vi "Loop_HW.vi"() -> ()   [LabVIEW 2017, in "LED Signal.lvlib"]
uses:
  LED Signal.lvlib
  Globals/Global_STOP.vi
  Global_SM_Data Out.vi
  ENUM_HW LED Commands.ctl
  Globals/Global_HW_Address_Assignments.vi
  <vilib>/Rock Robotics/WPI/SerialPort/WPI_SerialPortRef.ctl
  <vilib>/Rock Robotics/WPI/SerialPort/WPI_SerialPort.ctl
  Cluster_SM to HW Data.ctl
panel:
  out "SM LED_HW Cmd Data":T1
  out "SerialPortRef":T4
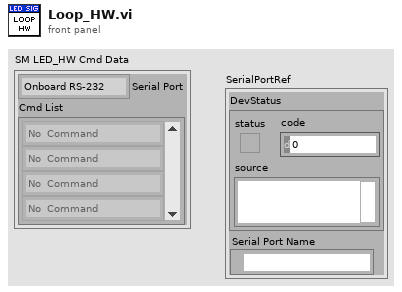
[diagram p1: front panel]
types:
  T1 = typedef "LED Signal.lvlib/Cluster_SM to HW Data.ctl" = cluster{"Serial Port":T2, "Cmd List":T3[]}
  T2 = typedef "WPI_SerialPort.ctl" = enum16{"Onboard RS-232", "MXP TTL", "USB 1", "USB 2"}
  T3 = typedef "LED Signal.lvlib/ENUM_HW LED Commands.ctl" = enum16{"No  Command", "Angled Drive; A", "Field Oriented Drive; D", "Normal Drive; d", "Camera Lined Up; C", "Camera Misallined; c", "Balls in Hopper; B", "Hopper Empty; b"}
  T4 = typedef "WPI_SerialPortRef.ctl" = cluster{"DevStatus":errorcluster, "Serial Port Name":refnum<visa-resource-name>}
  T5 = cluster{"Serial Port":T2, "Baud Rate":u32, "Data Bits":u16, "Parity":u16, "Stop Bits":u16, "Flow Control":u16}
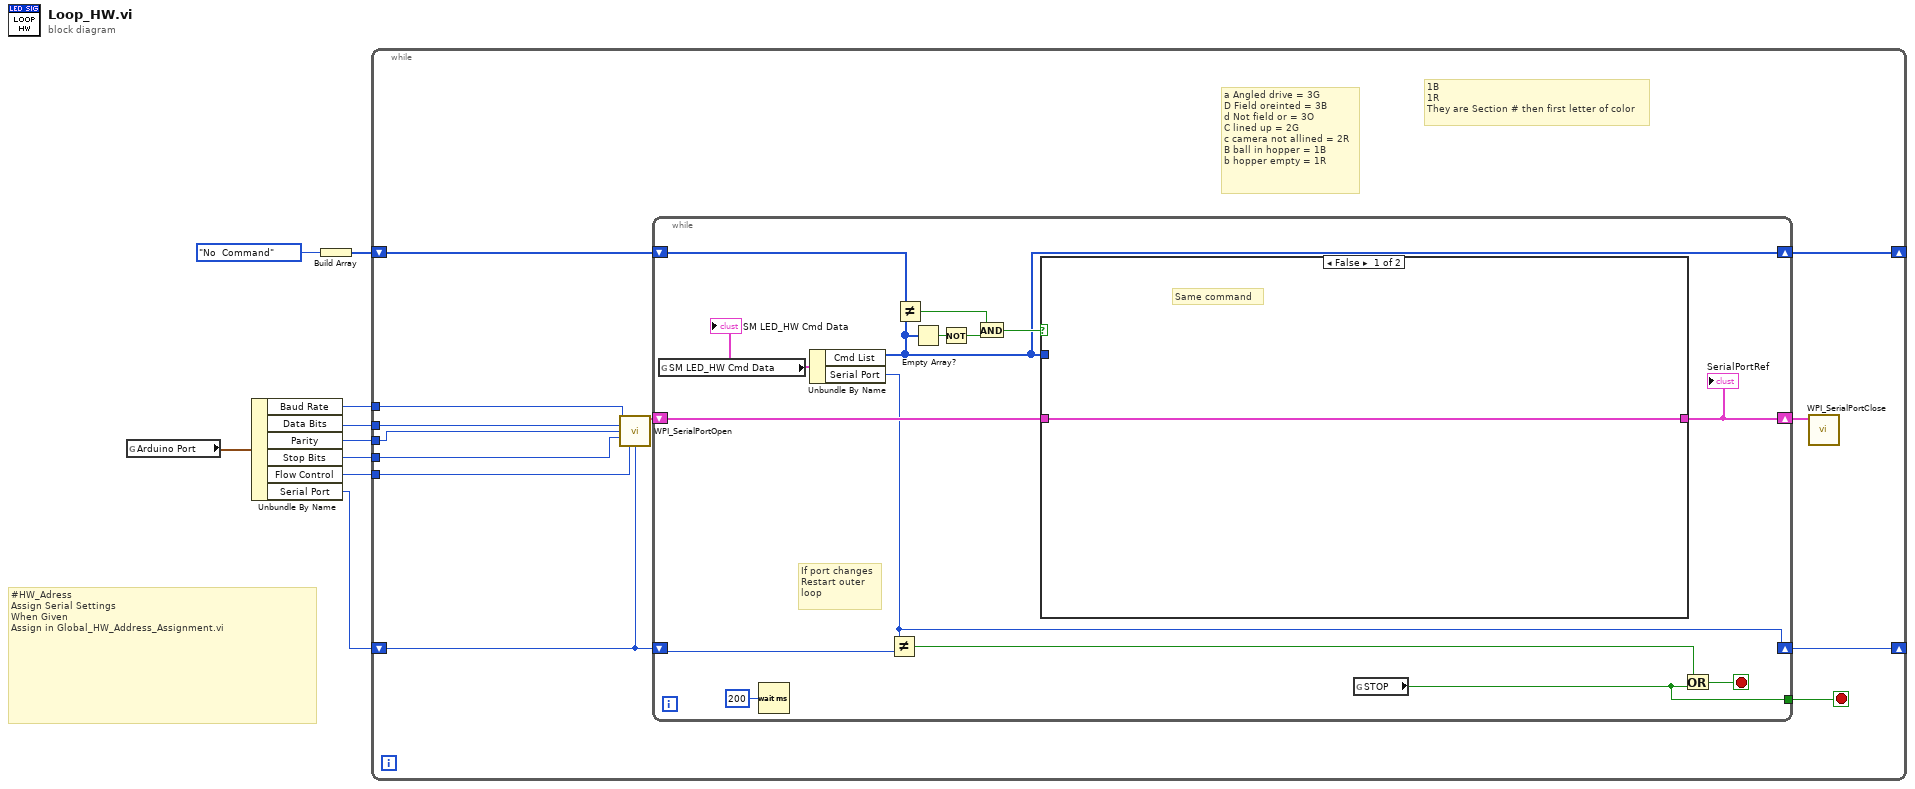
[diagram p0: block diagram]
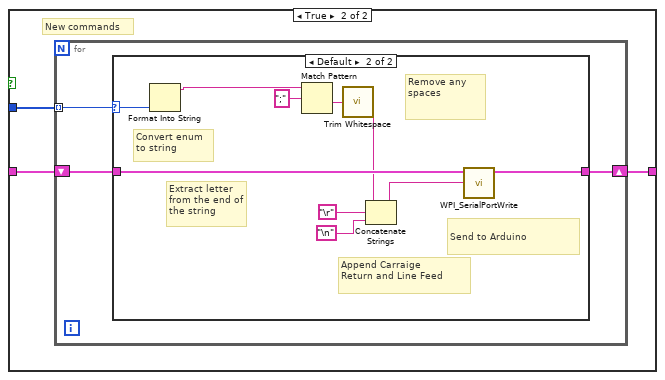
[diagram p2: hidden frame]
diagram:
  # "#HW_Adress\nAssign Serial Settings\nWhen Given\nAssign in Global_HW_Address_Assignment.vi"
  n1 = global read "Global_HW_Address_Assignments.vi" "Arduino Port"() -> (w7:T5)
  n2 = Unbundle By Name(w7) -> ("Baud Rate"=w5:u32, "Data Bits"=w4:u16, "Parity"=w3:u16, "Stop Bits"=w2:u16, "Flow Control"=w1:u16, "Serial Port"=w6:T2)
  n3 = Build Array(ENUM_HW_LED_Commands."No  Command" ("Cmd")) -> (w8:T3[])
  n4 = while {
    shift-right: [w19] -> _
    shift-left: w8 -> [w18]
    shift-right: [w17] -> _
    shift-left: w6 -> [w16]
    tunnel: w5 -> [w14]
    tunnel: w4 -> [w13]
    tunnel: w3 -> [w12]
    tunnel: w2 -> [w11]
    tunnel: w1 -> [w10]
    stop <- w15 stop-if-true
    # "1B\n1R\nThey are Section # then first letter of color"
    # "a Angled drive = 3G\nD Field oreinted = 3B\nd Not field or = 3O\nC lined up = 2G\nc camera not allined = 2R\nB ball in hopper = 1B\nb hopper empty = 1R"
    n5 = call <vilib>:"WPI_SerialPortOpen.vi"("Baud Rate"=w14, "Data Bits"=w13, "Parity"=w12, "Stop Bits"=w11, "Flow Control"=w10, "Serial Port"=w16) -> ("SerialPortRef"=w21:T4)  [unwired: 8 in, 1 out]
    n6 = while {
      shift-right: [w35] -> w20
      shift-left: w21 -> [w36]
      shift-right: [w24] -> w19
      shift-left: w18 -> [w31]
      shift-right: [w30] -> w17
      shift-left: w16 -> [w29]
      tunnel: [w22] -> w15
      stop <- w34 stop-if-true
      # "If port changes\nRestart outer \nloop"
      n7 = global read "Global_SM_Data Out.vi" "SM LED_HW Cmd Data"() -> (w32:T1)
      "SM LED_HW Cmd Data" <- w32
      n8 = Wait (ms)(milliseconds to wait=u32 200) -> ()  [unwired: 1 out]
      n9 = Unbundle By Name(w32) -> ("Cmd List"=w24:T3[], "Serial Port"=w30:T2)
      n10 = Not Equal?(x=w30, y=w29) -> (x != y?=w28:bool)
      n11 = Not Equal?(x=w31, y=w24) -> (x != y?=w27:bool)
      n12 = Empty Array?(array=w24) -> (empty?=w25:bool)
      n13 = Not(x=w25) -> (.not. x?=w23:bool)
      n14 = And(x=w27, y=w23) -> (x .and. y?=w26:bool)
      n15 = case shown="False" w26 {
        tunnel: w36 -> [w37 w40]
        tunnel: [w37 w39] -> w35
        tunnel: w24 -> [_ w38]
        frame False {
          # "Same command"
        }
        frame True {
          # "New commands"
          n16 = for {
            tunnel: w38 -> [w41] mode=indexing
            shift-right: [w42] -> w39
            shift-left: w40 -> [w43]
            n17 = case shown="Default" w41 {
              selector: w41 -> [_ w49]
              tunnel: w43 -> [w44 w54]
              tunnel: [w44 w50] -> w42
              frame "No  Command" {
              }
              frame Default {
                # "Send to Arduino"
                # "Append Carraige \nReturn and Line Feed"
                # "Remove any\nspaces"
                # "Extract letter \nfrom the end of the string"
                # "Convert enum\nto string"
                n18 = Format Into String(w49) -> (resulting string=w48:string)  [unwired: 3 in, 1 out]
                n19 = Match Pattern(string=w48, regular expression=";") -> (after substring=w46:string)  [unwired: 1 in, 3 out]
                n20 = call <vilib>:"Trim Whitespace.vi"("string"=w46) -> ("trimmed string"=w45:string)  [unwired: 1 in]
                n21 = Concatenate Strings(w45, "\r", "\n") -> (w51:string)
                n22 = call <vilib>:"WPI_SerialPortWrite.vi"("Buffer"=w51, "SerialPortRef"=w54) -> ("SerialPortRef"=w50:T4)  [unwired: 7 in, 2 out]
              }
            }
          }
        }
      }
      "SerialPortRef" <- w35
      n23 = global read "Global_STOP.vi" "STOP"() -> (w22:bool)
      n24 = Or(x=w28, y=w22) -> (x .or. y?=w34:bool)
    }
    n25 = call <vilib>:"WPI_SerialPortClose.vi"("SerialPortRef"=w20) -> ()  [unwired: 10 in, 1 out]
  }
